vi "Lead_2_DTF.vi"(8 "error in (no error)":errorcluster, 10 "Sampling Time [s]":dbl, 11 "Lead params":T2={"f_lead [Hz]"=0.0, "alpha"=10.0}) -> (0 "error out":errorcluster, 3 "TF model":T1 {"Denominator" format="%#.15g"; "Numerator" format="%#.15g"})   [LabVIEW 2020, in "PC-RT_Controller.lvlib"]
doc: "Convert lead with low-pass filter parameters (f_lead [Hz], alpha) into discrete-time transfer function model using Bilinear (tustin) transform."
uses:
  PC-RT_Controller.lvlib
  TypeDefs/Lead params.ctl
  TypeDefs/TF_model.ctl
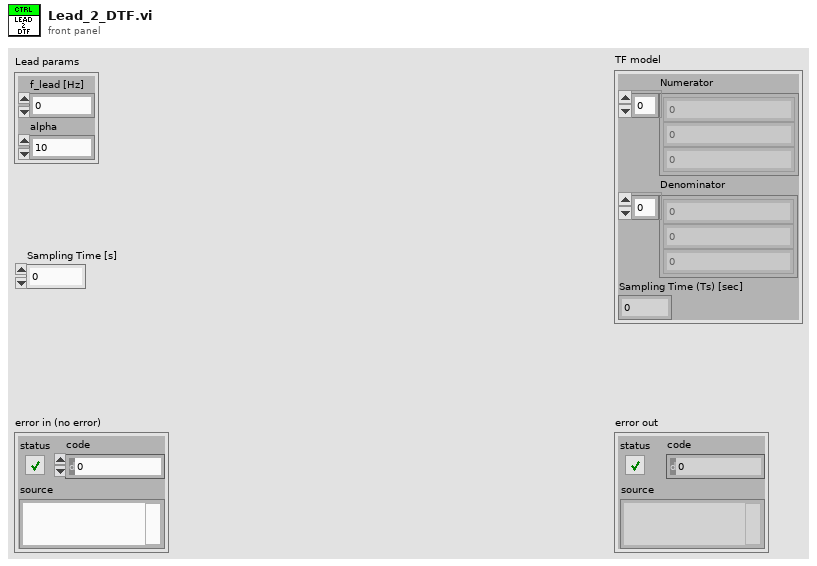
[diagram p1: front panel]
types:
  T1 = typedef "PC-RT_Controller.lvlib/TF_model.ctl" = cluster{"Numerator":dbl[], "Denominator":dbl[], "Sampling Time (Ts) [sec]":dbl}
  T2 = typedef "PC-RT_Controller.lvlib/Lead params.ctl" = cluster{"f_lead [Hz]":dbl, "alpha":dbl}
  T3 = typedef "PC-RT_Controller.lvlib/ZPK_model.ctl" = cluster{"Zero":cdb[], "Pole":cdb[], "Gain (K)":dbl, "Sampling Time (Ts) [sec]":dbl}
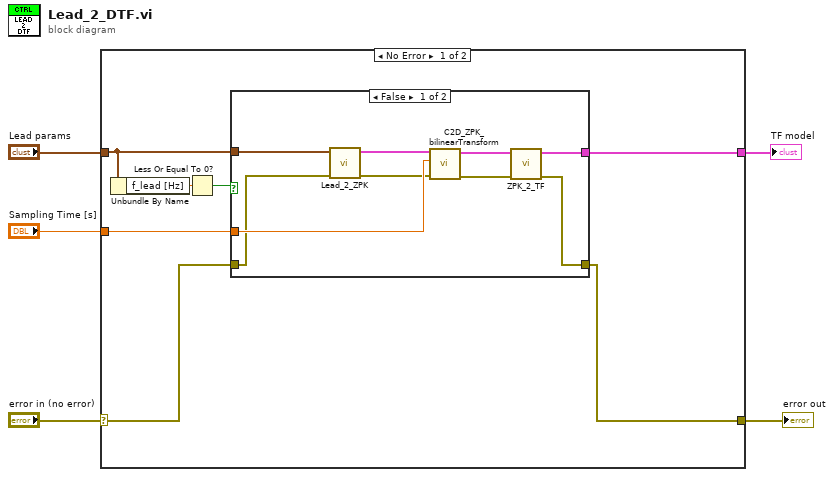
[diagram p0: block diagram]
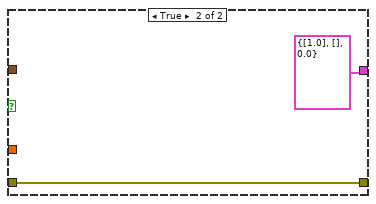
[diagram p2: hidden frame]
diagram:
  n1 = case shown="No Error" "error in (no error)" {
    selector: "error in (no error)" -> [w11 w24]
    tunnel: "Lead params" -> [w9 _]
    tunnel: [w6 w24] -> w3
    tunnel: "Sampling Time [s]" -> [w12 _]
    tunnel: [w10 _] -> w1
    frame No Error {
      n2 = Unbundle By Name(w9) -> ("f_lead [Hz]"=w8:dbl)
      n3 = Less Or Equal To 0?(x=w8) -> (x <= 0?=w7:bool)
      n4 = case shown="False" w7 {
        tunnel: w9 -> [w21 _]
        tunnel: w12 -> [w19 _]
        tunnel: w11 -> [w15 w22]
        tunnel: [w14 T1 {"Numerator"=[1.0], "Denominator"=[], "Sampling Time (Ts) [sec]"=0.0} ("TF model")] -> w10
        tunnel: [w13 w22] -> w6
        frame False {
          n5 = call "Lead_2_ZPK.vi"("error in (no error)"=w15, "Lead params"=w21) -> ("error out"=w17:errorcluster, "ZPK model"=w20:T3)  [unwired: 8 in]
          n6 = call "C2D_ZPK_bilinearTransform.vi"("error in (no error)"=w17, "Sampling Time (Ts) [s]"=w19, "ZPK model (CT)"=w20) -> ("error out"=w16:errorcluster, "ZPK model (DT)"=w18:T3)  [unwired: 7 in]
          n7 = call "ZPK_2_TF.vi"("error in (no error)"=w16, "ZPK model"=w18) -> ("error out"=w13:errorcluster, "TF model"=w14:T1)  [unwired: 8 in]
        }
        frame True {
        }
      }
    }
    frame Error {
    }
  }
  "error out" <- w3
  "TF model" <- w1
